vi "ExplorerDemo.vi"() -> ()   [LabVIEW 2018]
doc: "Use this template to build a user interface event handler design pattern. Use this pattern for dialog boxes and other user interfaces. You also can create and execute user-defined events that the VI can handle the same way as user interface events."
panel:
  out "error out":errorcluster
  out "x+1":i32
  out "data out":string
  in  "Button 1":bool
  in  "stop":bool
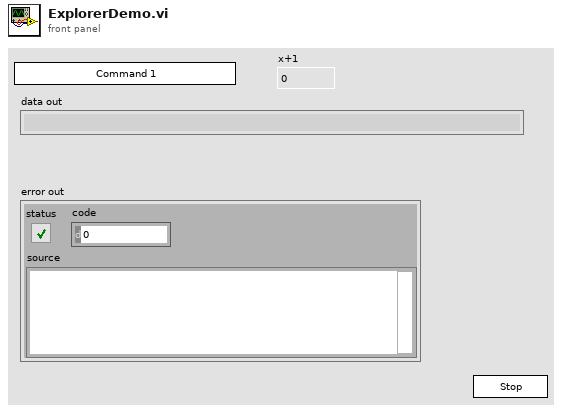
[diagram p1: front panel]
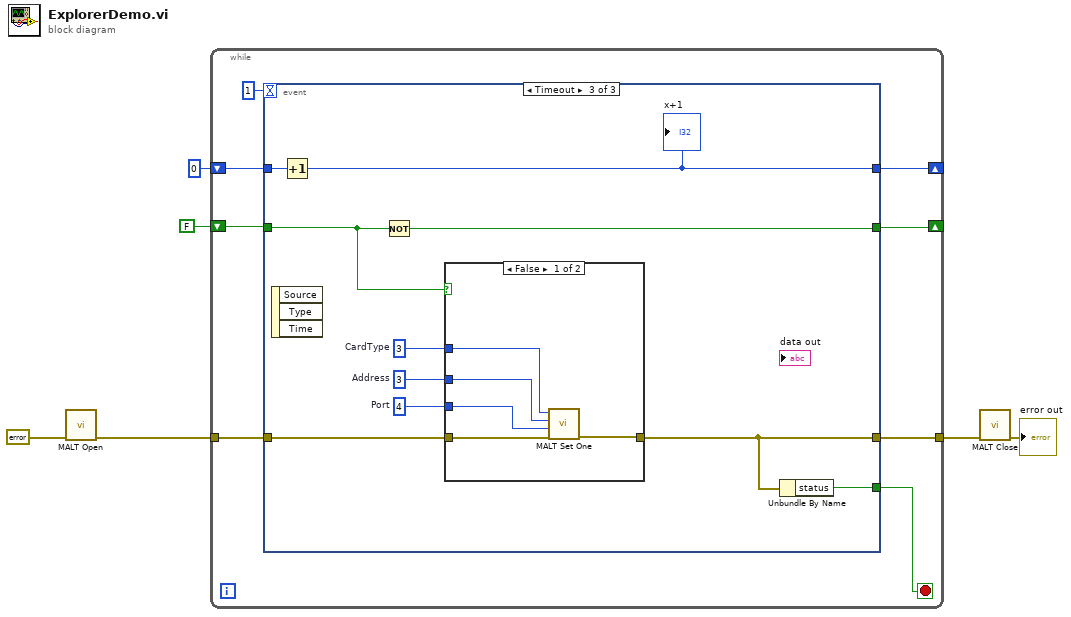
[diagram p0: block diagram]
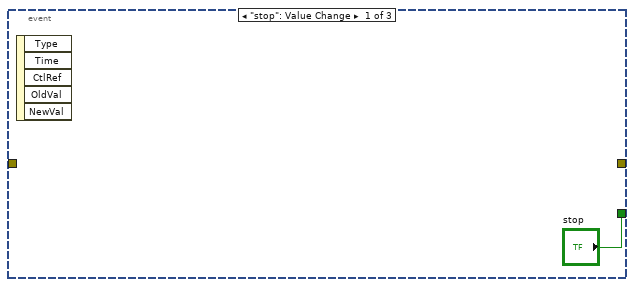
[diagram p2: hidden frame]
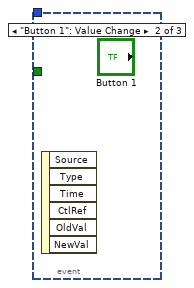
[diagram p3: hidden frame]
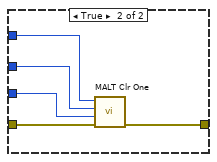
[diagram p4: hidden frame]
diagram:
  n1 = call "MALT Open.vi"("error in"=errorcluster {"status"=FALSE, "code"=0, "source"=""}) -> ("error out"=w4:errorcluster)  [unwired: 10 in]
  n2 = while {
    shift-right: [w12] -> _
    shift-left: FALSE -> [w11]
    tunnel: w4 -> [w10]
    shift-right: [w8] -> _
    shift-left: 0 -> [w9]
    tunnel: [w7] -> w2
    stop <- w14 stop-if-true
    n3 = event shown="[2] Timeout" {
      selector: _ -> [_ _ _]
      dyn-events: _ -> [_ _ _]
      timeout: 1 -> [_ _ _]
      tunnel: ["stop" _ w16] -> w14
      tunnel: w11 -> [_ _ w23]
      tunnel: [_ _ w22] -> w12
      tunnel: w10 -> [_ _ w21]
      tunnel: w9 -> [_ _ w25]
      tunnel: [_ _ w24] -> w8
      tunnel: [_ _ w20] -> w7
      event "stop": Value Change {
        n4 = event-data() -> ()  [unwired: 1 in, 5 out]
      }
      event "Button 1": Value Change {
        n5 = event-data() -> ()  [unwired: 1 in, 6 out]
      }
      event Timeout {
        w17 = 3  # CardType
        w18 = 3  # Address
        w19 = 4  # Port
        n6 = event-data() -> ()  [unwired: 1 in, 3 out]
        n7 = Increment(x=w25) -> (x+1=w24:i32)
        "x+1" <- w24
        n8 = Not(x=w23) -> (.not. x?=w22:bool)
        n9 = case shown="False" w23 {
          tunnel: w21 -> [w30 w35]
          tunnel: [w29 w34] -> w20
          tunnel: w19 -> [w26 w33]
          tunnel: w18 -> [w27 w32]
          tunnel: w17 -> [w28 w31]
          frame False {
            n10 = call "MALT Set One.vi"("error in"=w30, "port"=w26, "address"=w27, "cardType"=w28) -> ("error out"=w29:errorcluster)  [unwired: 7 in]
          }
          frame True {
            n11 = call "MALT Clr One.vi"("error in"=w35, "port"=w33, "address"=w32, "cardType"=w31) -> ("error out"=w34:errorcluster)  [unwired: 7 in]
          }
        }
        n12 = Unbundle By Name(w20) -> ("status"=w16:bool)
      }
    }
  }
  n13 = call "MALT Close.vi"("error in"=w2) -> ("error out"=→"error out":errorcluster)  [unwired: 10 in]
